vi "Sender UI.vi"(8 "Error In":errorcluster, 10 "Message Data":string(combo)) -> (0 "Error Out":errorcluster)   [LabVIEW 2023, in "User Sender.lvclass"]
uses:
  User Sender.lvclass
  Controls/Message Type.ctl
  Controls/Queue Operation.ctl
  Controls/User Event Operations.ctl
  Controls/Messenger Data.ctl
  Message Type/Message Type.lvclass
  Controls/Type Class Ref.ctl
  Controls/Class DVR Ref.ctl
  Message Data/Message Data.lvclass
  User Sender.lvclass/User Sender.ctl
panel:
  in  "Calling Mode":string(combo)
  in  "Message Type":T1
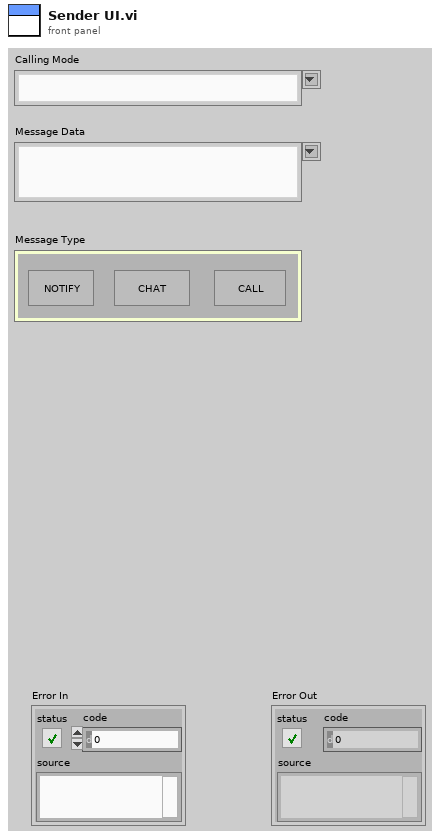
[diagram p1: front panel]
types:
  T1 = typedef "Message Type.ctl" = cluster{"Notify Only":bool, "Notify with Message":bool, "Stream":bool}
  T2 = typedef "Messenger Data.ctl" = cluster{"Message Data path":path, "Start Time":dbl, "Elapsed TIme":dbl, "Message Type":refnum<class "Message Type.lvclass">, "Selected Message Data":string, "Selected Message Type":string, "Type DVR Ref":T3[], "Data DVR Ref":T4[], "Type DVR":refnum<data-value>, "Data DVR":refnum<data-value>, "Stream?":bool}
  T3 = typedef "Type Class Ref.ctl" = cluster{"Class Name":string, "Class DVR Ref":refnum<data-value>}
  T4 = typedef "Class DVR Ref.ctl" = cluster{"Class DVR Ref":refnum<data-value>, "Class Name":string}
  T5 = typedef "User Event Operations.ctl" = enum16{"Obtain", "Generate", "Destroy"}
  T6 = typedef "Queue Operation.ctl" = enum16{"Create & Enqueue N", "Enqueue N", "Dequeue", "Enstack N", "Flush", "Release"}
  T7 = typedef "Queue Element.ctl" = cluster{"State":string, "Data":variant}
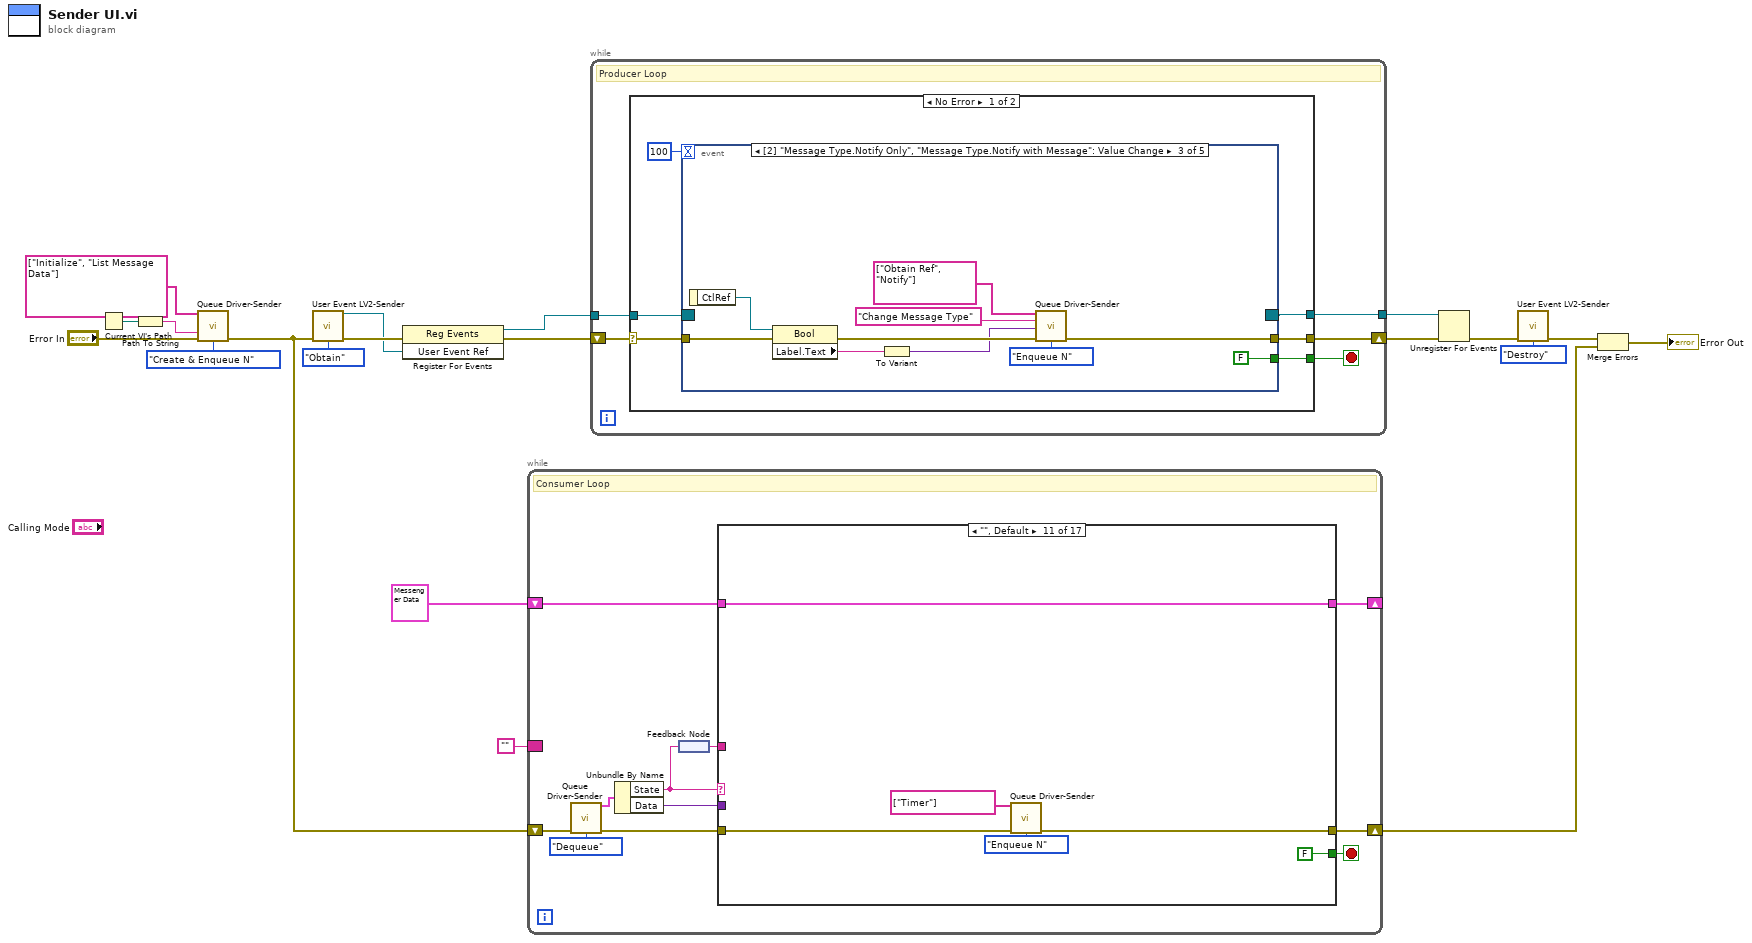
[diagram p0: block diagram]
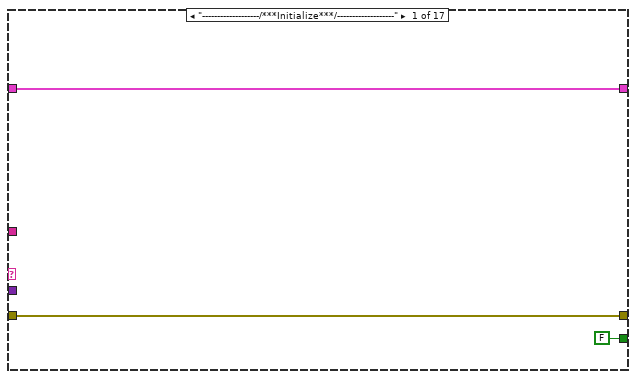
[diagram p2: hidden frame]
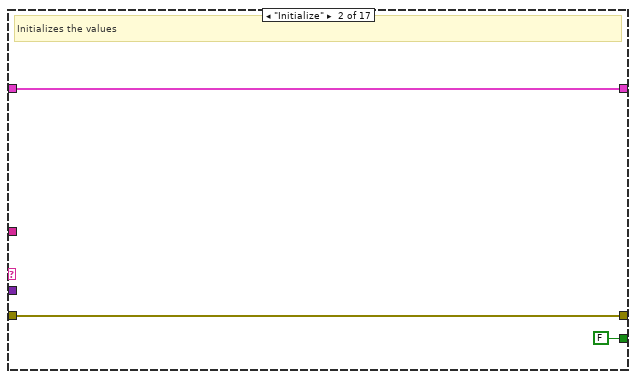
[diagram p3: hidden frame]
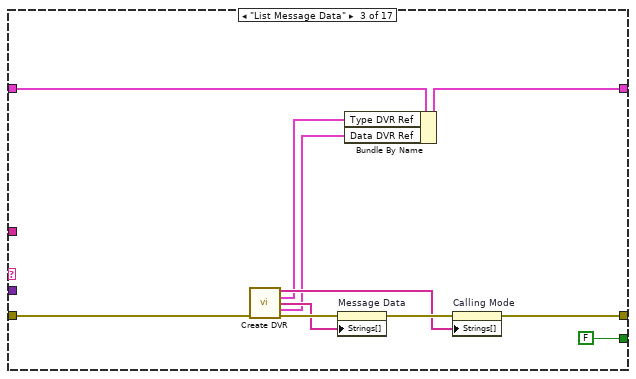
[diagram p4: hidden frame]
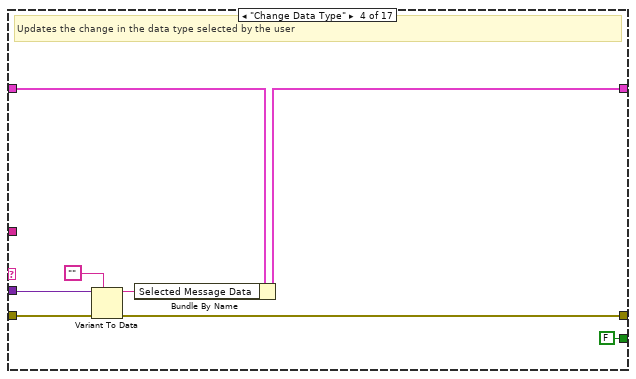
[diagram p5: hidden frame]
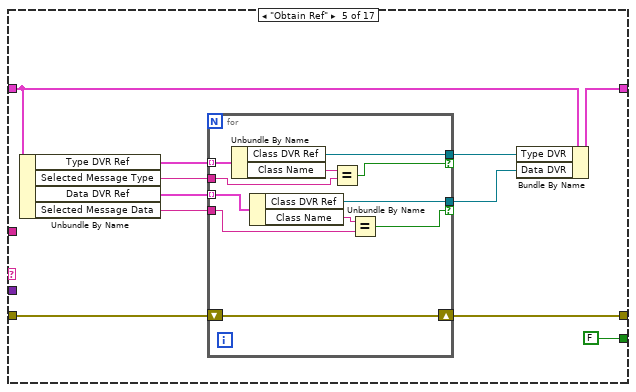
[diagram p6: hidden frame]
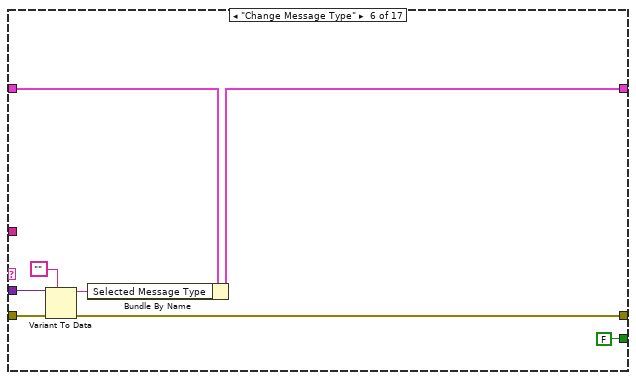
[diagram p7: hidden frame]
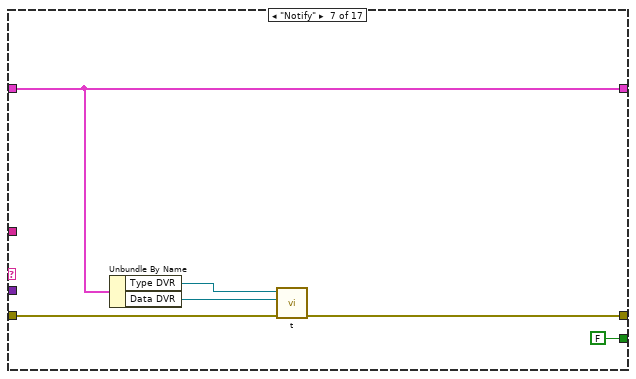
[diagram p8: hidden frame]
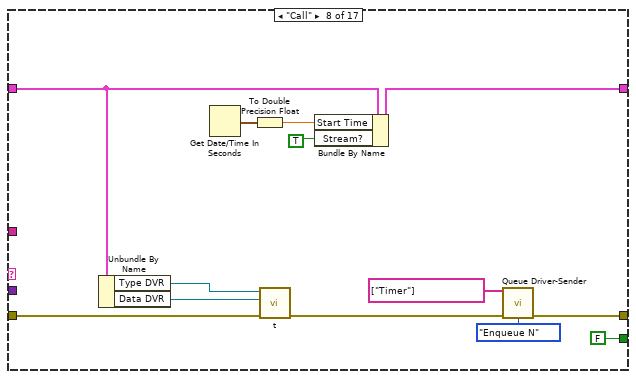
[diagram p9: hidden frame]
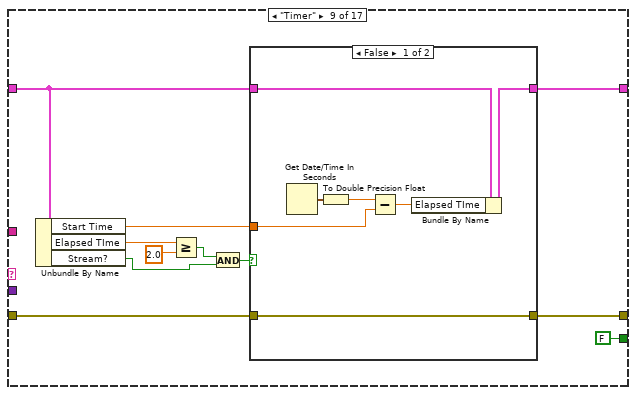
[diagram p10: hidden frame]
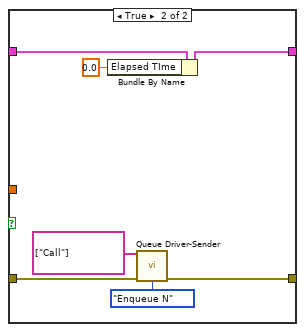
[diagram p11: hidden frame]
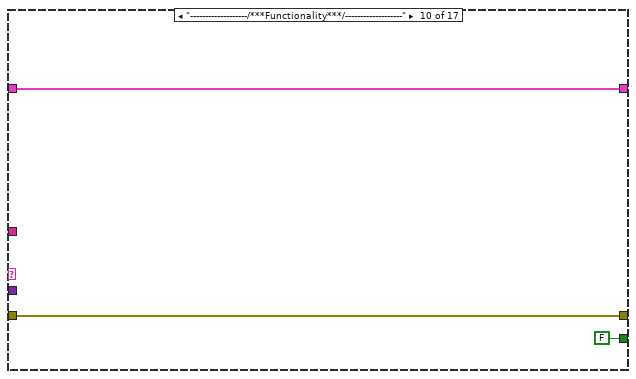
[diagram p12: hidden frame]
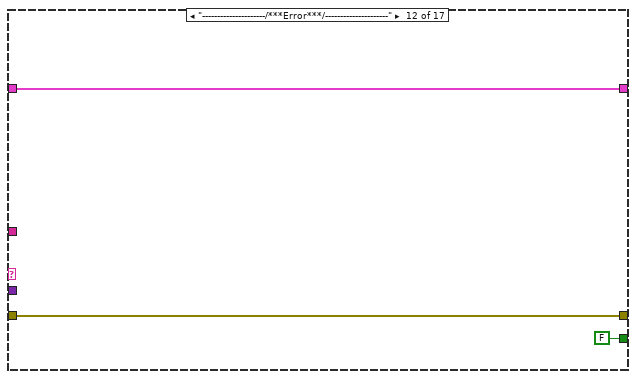
[diagram p13: hidden frame]
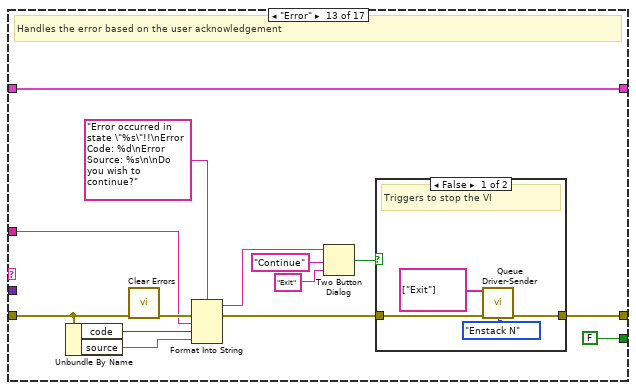
[diagram p14: hidden frame]
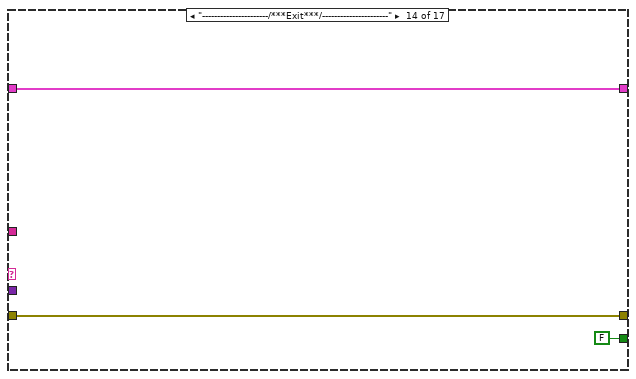
[diagram p16: hidden frame]
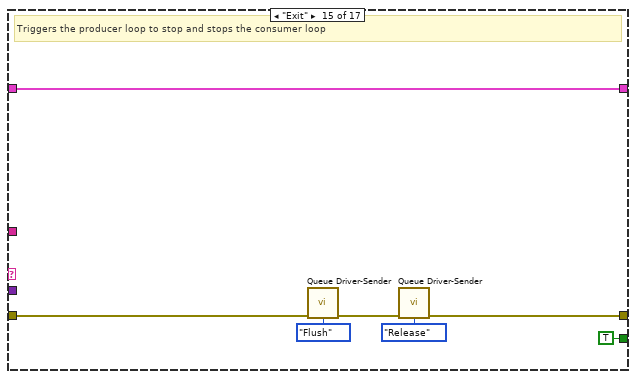
[diagram p17: hidden frame]
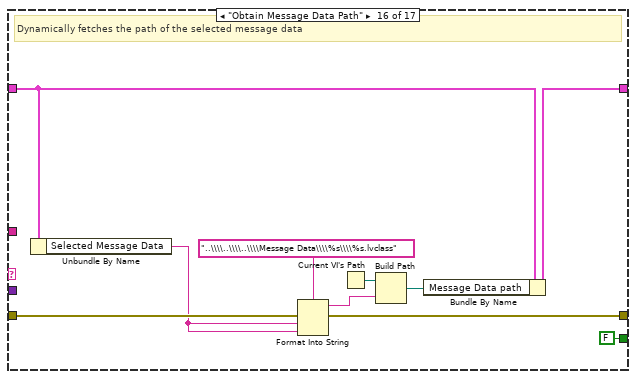
[diagram p18: hidden frame]
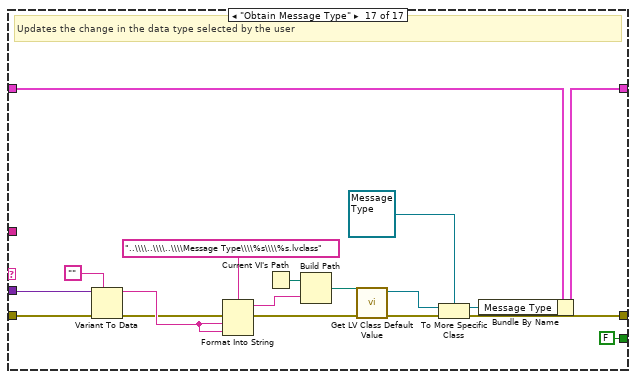
[diagram p19: hidden frame]
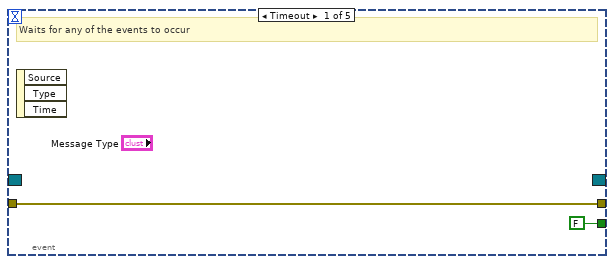
[diagram p20: hidden frame]
diagram:
  n1 = Current VI's Path() -> (path=w17:path)
  n2 = Path To String(path=w17) -> (string=w16:string)
  n3 = call "Queue Driver-Sender.vi"("States[]"=string[] ["Initialize", "List Message Data"], "Queue Name"=w16, "Error In"="Error In", "Queue Operation"=Queue_Operation."Create & Enqueue N") -> ("Error Out"=w10:errorcluster)  [unwired: 10 in, 1 out]
  n4 = call "User Event LV2-Sender.vi"("Error In"=w10, "Operation"=User_Event_Operations."Obtain") -> ("User Event Ref"=w8:refnum<user-event>, "Error Out"=w12:errorcluster)  [unwired: 12 in]
  n5 = register-events(error in=w12, w8) -> (reference out=w7:refnum<event-registration>, error out=w9:errorcluster)  [unwired: 1 in]
  n6 = while {
    shift-right: [w30] -> w13
    shift-left: w10 -> [w31]
    border: "" -> [_]
    shift-right: [w21] -> _
    shift-left: T2 {"Message Data path"=path "", "Start Time"=0.0, "Elapsed TIme"=0.0, "Message Type"=refnum, "Selected Message Data"="", "Selected Message Type"="", "Type DVR Ref"=[], "Data DVR Ref"=[], "Type DVR"=refnum, "Data DVR"=refnum, "Stream?"=FALSE} -> [w22]
    stop <- w26 stop-if-true
    # "Consumer Loop"
    n7 = call "Queue Driver-Sender.vi"("Error In"=w31, "Queue Operation"=Queue_Operation."Dequeue") -> ("Dequeue Element"=w27:T7, "Error Out"=w29:errorcluster)  [unwired: 12 in]
    n8 = Unbundle By Name(w27) -> ("State"=w25:string, "Data"=w23:variant)
    n9 = feedback-in #1(w25) -> ()
    n10 = feedback #1() -> (w24:string)
    n11 = case shown="\"\", Default" w25 {
      tunnel: w29 -> [w34 w36 w48 w56 w67 w86 w92 w105 w116 w133 w139 w142 w148 w164 w171 w181 w199]
      tunnel: [w34 w36 w42 w50 w66 w84 w90 w99 w114 w133 w136 w142 w145 w164 w167 w175 w190] -> w30
      tunnel: [FALSE FALSE FALSE FALSE FALSE FALSE FALSE FALSE FALSE FALSE FALSE FALSE FALSE FALSE TRUE FALSE FALSE] -> w26
      tunnel: w24 -> [_ _ _ _ _ _ _ _ _ _ _ _ w146 _ _ _ _]
      tunnel: w23 -> [_ _ _ w51 _ w83 _ _ _ _ _ _ _ _ _ _ w194]
      tunnel: w22 -> [w32 w35 w45 w53 w65 w85 w89 w96 w112 w131 w137 w140 w143 w162 w165 w174 w196]
      tunnel: [w32 w35 w40 w52 w59 w81 w89 w102 w111 w131 w137 w140 w143 w162 w165 w179 w195] -> w21
      frame "-------------------/***Initialize***/-------------------" {
      }
      frame "Initialize" {
        # "Initializes the values"
      }
      frame "List Message Data" {
        n12 = call "Create DVR.vi"("Error In"=w48) -> ("message type classes"=w41:string[], "Type DVR Ref"=w39:T3[], "Message data classes"=w43:string[], "Data DVR Ref"=w38:T4[], "Error Out"=w44:errorcluster)  [unwired: 10 in]
        n13 = property on="Message Data" class="CmbBox"(error in=w44, "Strings[]"=w43) -> (error out=w46:errorcluster)  [unwired: 1 in, 1 out]
        n14 = Bundle By Name(cluster=w45, "Type DVR Ref"=w39, "Data DVR Ref"=w38) -> (w40:T2)
        n15 = property on="Calling Mode" class="CmbBox"(error in=w46, "Strings[]"=w41) -> (error out=w42:errorcluster)  [unwired: 1 in, 1 out]
      }
      frame "Change Data Type" {
        # "Updates the change in the data type selected by the user"
        n16 = Variant To Data(error in=w56, type="", Variant=w51) -> (data=w49:string, error out=w50:errorcluster)
        n17 = Bundle By Name(cluster=w53, "Selected Message Data"=w49) -> (w52:T2)
      }
      frame "Obtain Ref" {
        n18 = Unbundle By Name(w65) -> ("Type DVR Ref"=w63:T3[], "Selected Message Type"=w62:string, "Data DVR Ref"=w64:T4[], "Selected Message Data"=w61:string)
        n19 = for {
          shift-right: [w78] -> w66
          shift-left: w67 -> [w78]
          tunnel: w64 -> [w72] mode=indexing
          tunnel: w63 -> [w77] mode=indexing
          tunnel: w62 -> [w75]
          tunnel: w61 -> [w69]
          tunnel: [w74] -> w58 if=w73
          tunnel: [w71] -> w57 if=w68
          n20 = Unbundle By Name(w77) -> ("Class DVR Ref"=w74:refnum<data-value>, "Class Name"=w76:string)
          n21 = Unbundle By Name(w72) -> ("Class DVR Ref"=w71:refnum<data-value>, "Class Name"=w70:string)
          n22 = Equal?(x=w76, y=w75) -> (x = y?=w73:bool)
          n23 = Equal?(x=w70, y=w69) -> (x = y?=w68:bool)
        }
        n24 = Bundle By Name(cluster=w65, "Type DVR"=w58, "Data DVR"=w57) -> (w59:T2)
      }
      frame "Change Message Type" {
        n25 = Variant To Data(error in=w86, type="", Variant=w83) -> (data=w80:string, error out=w84:errorcluster)
        n26 = Bundle By Name(cluster=w85, "Selected Message Type"=w80) -> (w81:T2)
      }
      frame "Notify" {
        n27 = Unbundle By Name(w89) -> ("Type DVR"=w88:refnum<data-value>, "Data DVR"=w87:refnum<data-value>)
        n28 = call "t.vi"("error in (no error)"=w92, "Data DVR"=w87, "Type DVR"=w88) -> ("error out"=w90:errorcluster)  [unwired: 8 in]
      }
      frame "Call" {
        n29 = Unbundle By Name(w96) -> ("Type DVR"=w95:refnum<data-value>, "Data DVR"=w94:refnum<data-value>)
        n30 = Get Date/Time In Seconds() -> (seconds since 1Jan1904=w100:timestamp)
        n31 = To Double Precision Float(number=w100) -> (double precision float=w101:dbl)
        n32 = call "t.vi"("error in (no error)"=w105, "Data DVR"=w94, "Type DVR"=w95) -> ("error out"=w103:errorcluster)  [unwired: 8 in]
        n33 = Bundle By Name(cluster=w96, "Start Time"=w101, "Stream?"=TRUE) -> (w102:T2)
        n34 = call "Queue Driver-Sender.vi"("States[]"=string[] ["Timer"], "Error In"=w103, "Queue Operation"=Queue_Operation."Enqueue N") -> ("Error Out"=w99:errorcluster)  [unwired: 11 in, 1 out]
      }
      frame "Timer" {
        n35 = Unbundle By Name(w112) -> ("Start Time"=w113:dbl, "Elapsed TIme"=w109:dbl, "Stream?"=w107:bool)
        n36 = Greater Or Equal?(x=w109, y=2.0) -> (x >= y?=w108:bool)
        n37 = And(x=w108, y=w107) -> (x .and. y?=w106:bool)
        n38 = case shown="False" w106 {
          tunnel: w116 -> [w122 w130]
          tunnel: [w122 w128] -> w114
          tunnel: w113 -> [w117 _]
          tunnel: [w121 w125] -> w111
          tunnel: w112 -> [w123 w129]
          frame False {
            n39 = Get Date/Time In Seconds() -> (seconds since 1Jan1904=w120:timestamp)
            n40 = To Double Precision Float(number=w120) -> (double precision float=w118:dbl)
            n41 = Subtract(x=w118, y=w117) -> (x-y=w119:dbl)
            n42 = Bundle By Name(cluster=w123, "Elapsed TIme"=w119) -> (w121:T2)
          }
          frame True {
            n43 = Bundle By Name(cluster=w129, "Elapsed TIme"=0.0) -> (w125:T2)
            n44 = call "Queue Driver-Sender.vi"("States[]"=string[] ["Call"], "Error In"=w130, "Queue Operation"=Queue_Operation."Enqueue N") -> ("Error Out"=w128:errorcluster)  [unwired: 11 in, 1 out]
          }
        }
      }
      frame "-------------------/***Functionality***/-------------------" {
      }
      frame "", Default {
        n45 = call "Queue Driver-Sender.vi"("States[]"=string[] ["Timer"], "Error In"=w139, "Queue Operation"=Queue_Operation."Enqueue N") -> ("Error Out"=w136:errorcluster)  [unwired: 11 in, 1 out]
      }
      frame "---------------------/***Error***/---------------------" {
      }
      frame "Error" {
        # "Handles the error based on the user acknowledgement"
        n46 = Unbundle By Name(w148) -> ("code"=w150:i32, "source"=w149:string)
        n47 = call <vilib>:"Clear Errors.vi"("error in (no error)"=w148) -> ("error out"=w155:errorcluster)  [unwired: 5 in, 1 out]
        n48 = Format Into String(format string="Error occurred in state \"%s\"!!\nError Code: %d\nError Source: %s\n\nDo you wish to continue?", error in=w155, w146, w150, w149) -> (resulting string=w153:string, error out=w147:errorcluster)  [unwired: 1 in]
        n49 = Two Button Dialog(message=w153, 1:"Exit" ("F button name (\"Cancel\")"), 2:"Continue" ("T button name (\"OK\")")) -> (T button?=w144:bool)
        n50 = case shown="False" w144 {
          tunnel: w147 -> [w160 w161]
          tunnel: [w159 w161] -> w145
          frame False {
            # "Triggers to stop the VI"
            n51 = call "Queue Driver-Sender.vi"("States[]"=string[] ["Exit"], "Error In"=w160, "Queue Operation"=Queue_Operation."Enstack N") -> ("Error Out"=w159:errorcluster)  [unwired: 11 in, 1 out]
          }
          frame True {
          }
        }
      }
      frame "----------------------/***Exit***/----------------------" {
      }
      frame "Exit" {
        # "Triggers the producer loop to stop and stops the consumer loop"
        n52 = call "Queue Driver-Sender.vi"("Error In"=w171, "Queue Operation"=Queue_Operation."Flush") -> ("Error Out"=w169:errorcluster)  [unwired: 12 in, 1 out]
        n53 = call "Queue Driver-Sender.vi"("Error In"=w169, "Queue Operation"=Queue_Operation."Release") -> ("Error Out"=w167:errorcluster)  [unwired: 12 in, 1 out]
      }
      frame "Obtain Message Data Path" {
        # "Dynamically fetches the path of the selected message data"
        n54 = Unbundle By Name(w174) -> ("Selected Message Data"=w173:string)
        n55 = Format Into String(format string="..\\\\..\\\\..\\\\Message Data\\\\%s\\\\%s.lvclass", error in=w181, w173, w173) -> (resulting string=w177:string, error out=w175:errorcluster)  [unwired: 1 in]
        n56 = Current VI's Path() -> (path=w178:path)
        n57 = Build Path(base path=w178, name or relative path=w177) -> (appended path=w172:path)
        n58 = Bundle By Name(cluster=w174, "Message Data path"=w172) -> (w179:T2)
      }
      frame "Obtain Message Type" {
        # "Updates the change in the data type selected by the user"
        n59 = Variant To Data(error in=w199, type="", Variant=w194) -> (data=w185:string, error out=w184:errorcluster)
        n60 = Format Into String(format string="..\\\\..\\\\..\\\\Message Type\\\\%s\\\\%s.lvclass", error in=w184, w185, w185) -> (resulting string=w187:string, error out=w182:errorcluster)  [unwired: 1 in]
        n61 = Current VI's Path() -> (path=w188:path)
        n62 = Build Path(base path=w188, name or relative path=w187) -> (appended path=w183:path)
        n63 = call <vilib>:"Get LV Class Default Value.vi"("error in (no error)"=w182, "class path"=w183) -> ("error out"=w193:errorcluster, "object"=w192:refnum<class>)  [unwired: 8 in]
        n64 = To More Specific Class(target class=refnum<class "Message Type.lvclass"> refnum ("Message Type.lvclass"), reference=w192, error in=w193) -> (specific class reference=w189:refnum<class "Message Type.lvclass">, error out=w190:errorcluster)
        n65 = Bundle By Name(cluster=w196, "Message Type"=w189) -> (w195:T2)
      }
    }
  }
  n66 = while {
    shift-right: [w202] -> w19
    shift-left: w9 -> [w203]
    tunnel: w7 -> [w201]
    tunnel: [w200] -> w5
    stop <- w204 stop-if-true
    # "Producer Loop"
    n67 = case shown="No Error" w203 {
      selector: w203 -> [w209 w252]
      tunnel: [w210 FALSE] -> w204
      tunnel: [w208 w252] -> w202
      tunnel: w201 -> [w206 _]
      tunnel: [w205 _] -> w200
      frame No Error {
        n68 = event shown="[2] \"Message Type.Notify Only\", \"Message Type.Notify with Message\": Value Change" {
          selector: w206 -> [_ _ _ _ _]
          dyn-events: [_ _ _ _ _] -> w205
          timeout: 100 -> [_ _ _ _ _]
          tunnel: [FALSE w214 FALSE FALSE FALSE] -> w210
          tunnel: w209 -> [w211 w216 w233 w238 w250]
          tunnel: [w211 w215 w232 w243 w248] -> w208
          event Timeout {
            # "Waits for any of the events to occur"
            n69 = event-data() -> ()  [unwired: 1 in, 3 out]
          }
          event User Event {
            n70 = event-data() -> ("State"=w213:string)  [unwired: 1 in]
            n71 = case shown="\"False\", Default" w213 {
              tunnel: w216 -> [w218 w223]
              tunnel: [w218 w221] -> w215
              tunnel: [FALSE TRUE] -> w214
              frame "False", Default {
              }
              frame "Stop" {
                n72 = call "Queue Driver-Sender.vi"("States[]"=string[] ["Exit"], "Error In"=w223, "Queue Operation"=Queue_Operation."Enstack N") -> ("Error Out"=w221:errorcluster)  [unwired: 11 in, 1 out]
              }
            }
          }
          event Value Change {
            n73 = event-data() -> ("CtlRef"=w228:refnum<vi>)  [unwired: 1 in]
            n74 = property class="Bool"(reference=w228, error in=w233) -> (error out=w229:errorcluster, "Label.Text"=w225:string)  [unwired: 1 out]
            n75 = To Variant(anything=w225) -> (Variant=w224:variant)
            n76 = call "Queue Driver-Sender.vi"("States[]"=string[] ["Obtain Ref", "Notify"], "State"="Change Message Type", "Data"=w224, "Error In"=w229, "Queue Operation"=Queue_Operation."Enqueue N") -> ("Error Out"=w232:errorcluster)  [unwired: 9 in, 1 out]
          }
          event Value Change {
            n77 = event-data() -> ("CtlRef"=w234:refnum<vi>)  [unwired: 1 in]
            n78 = property class="Bool"(reference=w234, error in=w238) -> (error out=w237:errorcluster, "Label.Text"=w239:string)  [unwired: 1 out]
            n79 = To Variant(anything=w239) -> (Variant=w235:variant)
            n80 = call "Queue Driver-Sender.vi"("States[]"=string[] ["Obtain Ref", "Call"], "State"="Change Message Type", "Data"=w235, "Error In"=w237, "Queue Operation"=Queue_Operation."Enqueue N") -> ("Error Out"=w243:errorcluster)  [unwired: 9 in, 1 out]
          }
          event "Message Data": Value Change {
            n81 = event-data() -> ("NewVal"=w247:string)  [unwired: 1 in]
            n82 = To Variant(anything=w247) -> (Variant=w246:variant)
            n83 = call "Queue Driver-Sender.vi"("State"="Change Data Type", "Data"=w246, "Error In"=w250, "Queue Operation"=Queue_Operation."Enqueue N") -> ("Error Out"=w248:errorcluster)  [unwired: 10 in, 1 out]
          }
        }
      }
      frame Error {
      }
    }
  }
  n84 = Unregister For Events(event registration refnum=w5, error in=w19) -> (error out=w6:errorcluster)
  n85 = call "User Event LV2-Sender.vi"("Error In"=w6, "Operation"=User_Event_Operations."Destroy") -> ("Error Out"=w4:errorcluster)  [unwired: 12 in, 1 out]
  n86 = Merge Errors(w4, w13) -> (→"Error Out":errorcluster)
